vi "Build Description String.vi"(8 "error in (no error)":errorcluster, 11 "Boolean Assertion in":refnum<class "Boolean Assertion.lvclass">) -> (0 "error out":errorcluster, 2 "Description":string, 3 "Boolean Assertion out":refnum<class "Boolean Assertion.lvclass">)   [LabVIEW 2020, in "MacroAssert.lvlib" / "Boolean Assertion.lvclass"]
doc: "Builds a string to describe what <B>Step</B> does."
uses:
  Boolean Assertion.lvclass
  C:/Users/User/Documents/LabVIEW Data/Projects/MacroAssert/source/Classes/Assertion Step/Assertion Step.lvclass
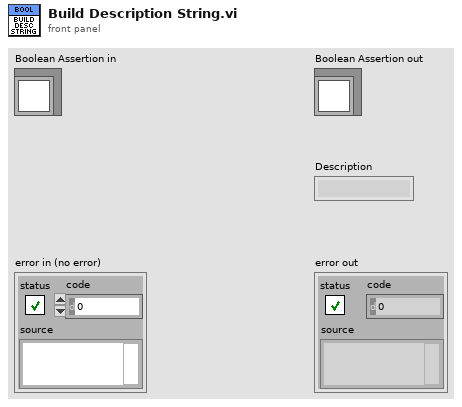
[diagram p1: front panel]
types:
  T1 = typedef "MacroAssert.lvlib/Boolean Assertion.lvclass/Boolean Assertion Type.ctl" = enum16{"Boolean Ctl Value", "Ctl Visible Property", "Ctl is Enabled", "Ctl is Grayed Out", "Ctl Key Focus Property", "Window is in Running Windows", "VI Front Panel is Open"}
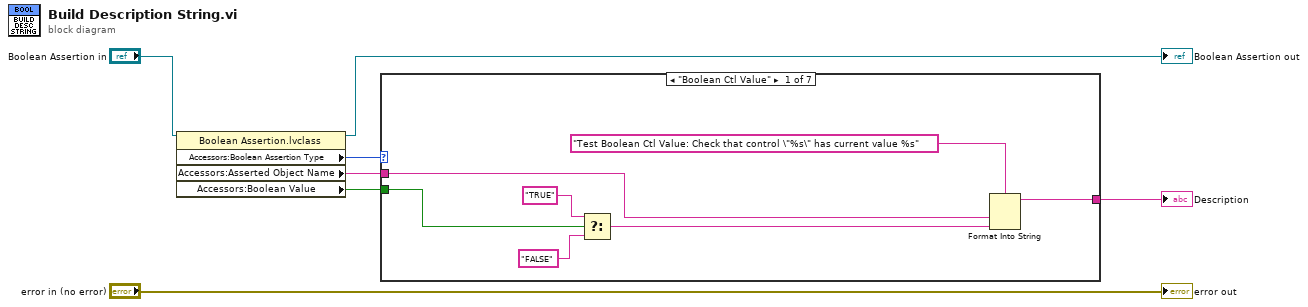
[diagram p0: block diagram]
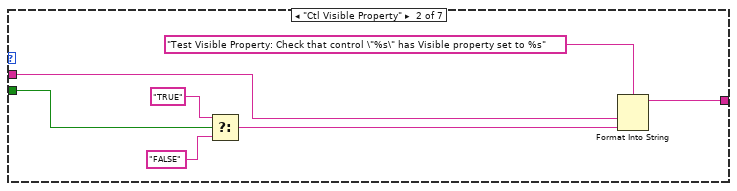
[diagram p2: hidden frame]
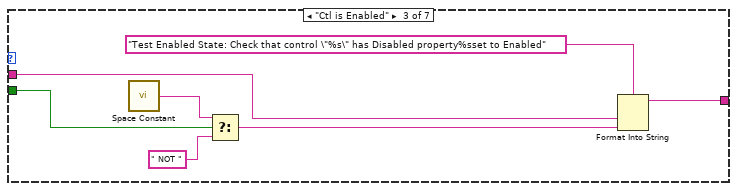
[diagram p3: hidden frame]
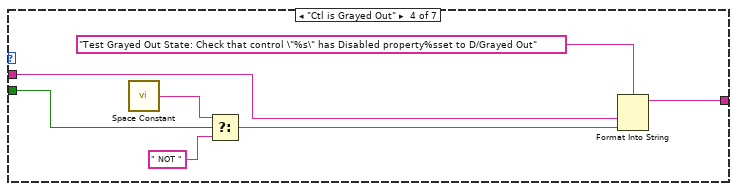
[diagram p4: hidden frame]
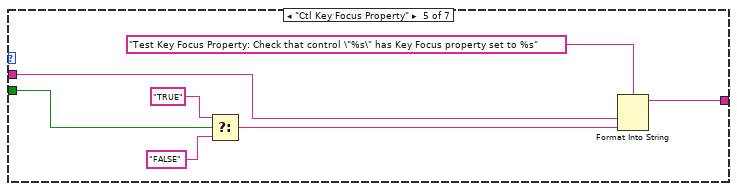
[diagram p5: hidden frame]
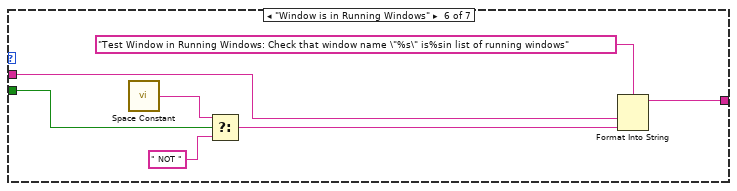
[diagram p6: hidden frame]
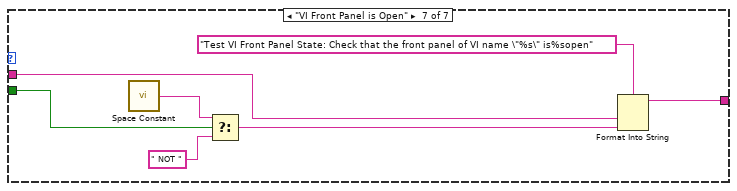
[diagram p7: hidden frame]
diagram:
  n1 = property class="Boolean Assertion.lvclass"(reference="Boolean Assertion in") -> (reference out=→"Boolean Assertion out":refnum<class "Boolean Assertion.lvclass">, "Accessors:Boolean Assertion Type"=w1:T1, "Accessors:Asserted Object Name"=w3:string, "Accessors:Boolean Value"=w4:bool)  [unwired: 1 in, 1 out]
  n2 = case shown="\"Boolean Ctl Value\"" w1 {
    tunnel: [w13 w20 w27 w34 w41 w48 w55] -> w5
    tunnel: w4 -> [w12 w19 w26 w33 w40 w47 w54]
    tunnel: w3 -> [w8 w15 w22 w29 w36 w43 w50]
    frame "Boolean Ctl Value" {
      n3 = Select(t="TRUE", s=w12, f="FALSE") -> (s? t:f=w9:string)
      n4 = Format Into String(format string="Test Boolean Ctl Value: Check that control \"%s\" has current value %s", w8, w9) -> (resulting string=w13:string)  [unwired: 2 in, 1 out]
    }
    frame "Ctl Visible Property" {
      n5 = Select(t="TRUE", s=w19, f="FALSE") -> (s? t:f=w16:string)
      n6 = Format Into String(format string="Test Visible Property: Check that control \"%s\" has Visible property set to %s", w15, w16) -> (resulting string=w20:string)  [unwired: 2 in, 1 out]
    }
    frame "Ctl is Enabled" {
      n7 = call <vilib>:"Space Constant.vi"() -> ("String"=w25:string)
      n8 = Select(t=w25, s=w26, f=" NOT ") -> (s? t:f=w23:string)
      n9 = Format Into String(format string="Test Enabled State: Check that control \"%s\" has Disabled property%sset to Enabled", w22, w23) -> (resulting string=w27:string)  [unwired: 2 in, 1 out]
    }
    frame "Ctl is Grayed Out" {
      n10 = call <vilib>:"Space Constant.vi"() -> ("String"=w32:string)
      n11 = Select(t=w32, s=w33, f=" NOT ") -> (s? t:f=w30:string)
      n12 = Format Into String(format string="Test Grayed Out State: Check that control \"%s\" has Disabled property%sset to D/Grayed Out", w29, w30) -> (resulting string=w34:string)  [unwired: 2 in, 1 out]
    }
    frame "Ctl Key Focus Property" {
      n13 = Select(t="TRUE", s=w40, f="FALSE") -> (s? t:f=w37:string)
      n14 = Format Into String(format string="Test Key Focus Property: Check that control \"%s\" has Key Focus property set to %s", w36, w37) -> (resulting string=w41:string)  [unwired: 2 in, 1 out]
    }
    frame "Window is in Running Windows" {
      n15 = call <vilib>:"Space Constant.vi"() -> ("String"=w46:string)
      n16 = Select(t=w46, s=w47, f=" NOT ") -> (s? t:f=w44:string)
      n17 = Format Into String(format string="Test Window in Running Windows: Check that window name \"%s\" is%sin list of running windows", w43, w44) -> (resulting string=w48:string)  [unwired: 2 in, 1 out]
    }
    frame "VI Front Panel is Open" {
      n18 = call <vilib>:"Space Constant.vi"() -> ("String"=w53:string)
      n19 = Select(t=w53, s=w54, f=" NOT ") -> (s? t:f=w51:string)
      n20 = Format Into String(format string="Test VI Front Panel State: Check that the front panel of VI name \"%s\" is%sopen", w50, w51) -> (resulting string=w55:string)  [unwired: 2 in, 1 out]
    }
  }
  "Description" <- w5
  "error out" <- "error in (no error)"
